vi "Demo WSGI.vi"() -> ()   [LabVIEW 2021, in "HttpServer.lvlib"]
uses:
  HttpServer.lvlib
  TypeDefs/WSGI.ctl
  <vilib>/Utility/error.llb/Error Cluster From Error Code.vi
  <vilib>/ErrorRing/Error Ring.xnode
panel:
  in  "Request":string="GET /log HTTP/1.1"
  out "Content":string
  out "Response Headers":map{string, string}(c390)
  out "Status":string
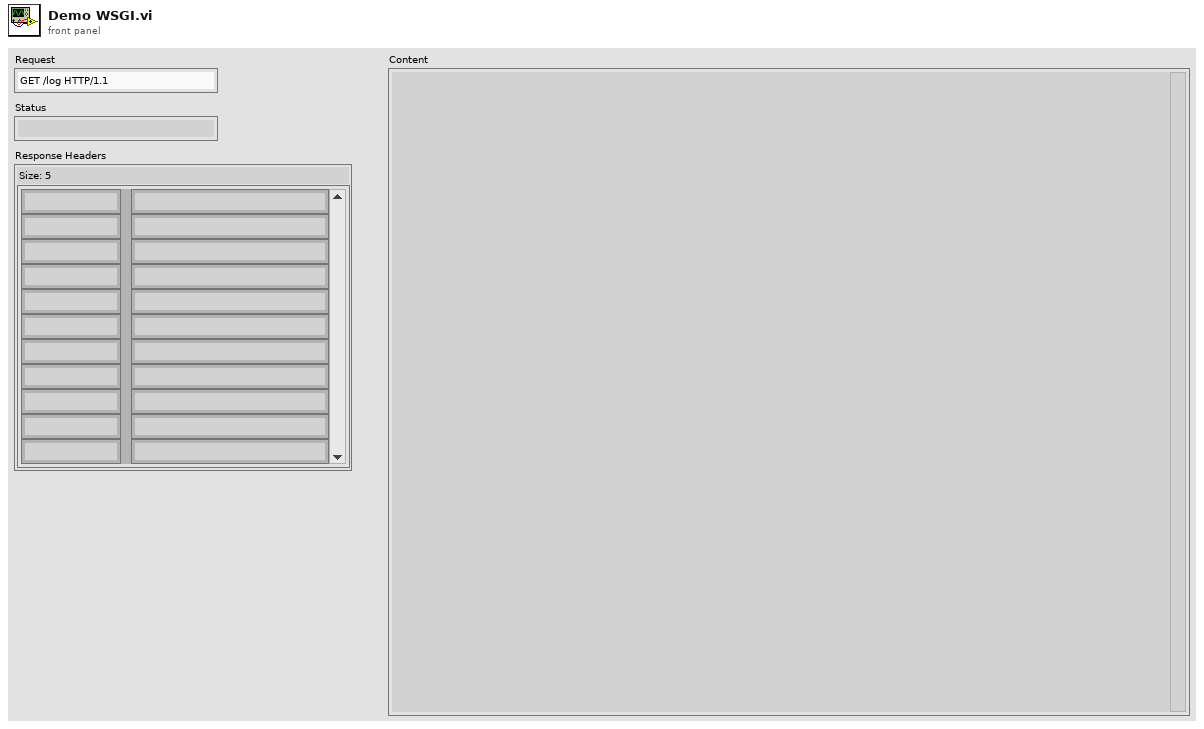
[diagram p1: front panel]
types:
  T1 = typedef "HttpServer.lvlib/WSGI.ctl" = cluster{"Header-Line":string, "Headers":map{string, string}, "Content":string}
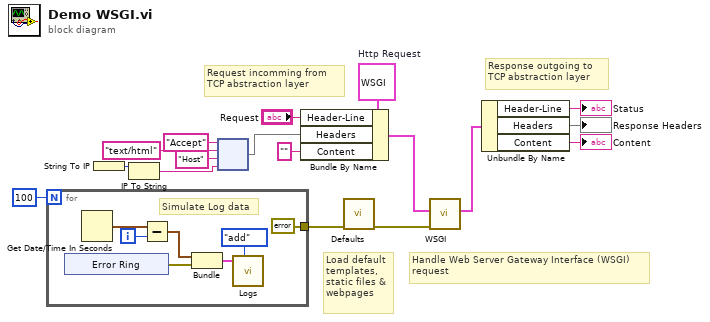
[diagram p0: block diagram]
diagram:
  w17 = T1 {"Header-Line"="", "Headers"={}, "Content"=""}  # Http Request
  # "Handle Web Server Gateway Interface (WSGI)\nrequest"
  # "Load default\ntemplates,\nstatic files &\nwebpages"
  # "Response outgoing to \nTCP abstraction layer"
  # "Request incomming from\nTCP abstraction layer"
  n1 = for {
    N: 100 -> [_]
    tunnel: [errorcluster {"status"=FALSE, "code"=0, "source"=""} ("error in (no error)")] -> w5
    i -> [w20]
    # "Simulate Log data"
    n2 = xnode "Error Ring"() -> ("error out"=w22:errorcluster)
    n3 = Get Date/Time In Seconds() -> (seconds since 1Jan1904=w19:timestamp)
    n4 = Subtract(x=w19, y=w20) -> (x-y=w18:timestamp)
    n5 = Bundle(w18, "error out"=w22) -> (w21:cluster{timestamp, "error out":errorcluster})  [unwired: 1 in]
    n6 = call "Logs.vi"("Action"=enum8{"noop", "add", "clear"}."add", "log"=w21) -> ()  [unwired: 9 in, 1 out]
  }
  n7 = String To IP() -> (0:w3:u32)  [unwired: 1 in]
  n8 = IP To String(2:w3) -> (0:w2:string)  [unwired: 1 in]
  n9 = node("Accept" ("key"), "text/html" ("key"), "Host" ("key"), w2) -> (w8:map{string, string})
  n10 = Bundle By Name(cluster=w17, "Header-Line"="Request", "Headers"=w8, "Content"="") -> (w12:T1)
  n11 = call "Defaults.vi"("error in (no error)"=w5) -> ("error out"=w6:errorcluster)  [unwired: 10 in]
  n12 = call "WSGI.vi"("error in (no error)"=w6, "WSGI Request"=w12) -> ("WSGI Response"=w16:T1)  [unwired: 8 in, 1 out]
  n13 = Unbundle By Name(w16) -> ("Header-Line"=→"Status":string, "Headers"=→"Response Headers":map{string, string}, "Content"=→"Content":string)
